vi "niDTS BT INSTR TX UTIL DataType and Rate.vi"(5 "Packet type":T2=enum."DH1", 7 "Data Rate":i32=1) -> (6 "Packet":T1={"PacketType"=enum."DH1", "PacketPayloadDatarate"=1})   [LabVIEW 2015, in "niDTS BT.lvlib" / "niDTS BT INSTR TX.lvclass"]
uses:
  niDTS BT INSTR TX.lvclass
  Includes/niDTS BT INC Packet Type.ctl
  niDTS BT.lvlib
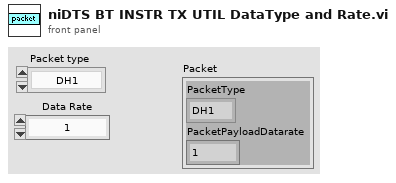
[diagram p1: front panel]
types:
  T1 = cluster{"PacketType":enum16{"DH1", "DH3", "DH5", "LETP"}, "PacketPayloadDatarate":i32}
  T2 = typedef "niDTS BT.lvlib/niDTS BT INC Packet Type.ctl" = enum16{"NULL", "POLL", "FHS", "DM1", "DH1", "HV1", "HV2", "HV3", "EV3", "DV", "AUX1", "DM3", "DH3", "EV4", "EV5", "DM5", "DH5", "LE-TP"}
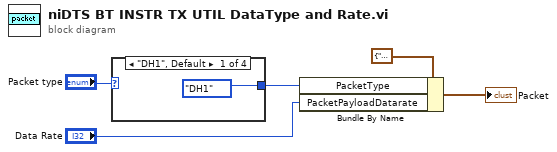
[diagram p0: block diagram]
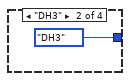
[diagram p2: hidden frame]
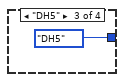
[diagram p3: hidden frame]
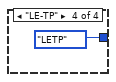
[diagram p4: hidden frame]
diagram:
  n1 = case shown="\"DH1\", Default" "Packet type" {
    tunnel: [enum16{"DH1", "DH3", "DH5", "LETP"}."DH1" ("PacketType") enum16{"DH1", "DH3", "DH5", "LETP"}."DH3" ("PacketType") enum16{"DH1", "DH3", "DH5", "LETP"}."DH5" ("PacketType") enum16{"DH1", "DH3", "DH5", "LETP"}."LETP" ("PacketType")] -> w2
    frame "DH1", Default {
    }
    frame "DH3" {
    }
    frame "DH5" {
    }
    frame "LE-TP" {
    }
  }
  n2 = Bundle By Name(cluster=T1 {"PacketType"=enum."DH1", "PacketPayloadDatarate"=1} ("Packet"), "PacketType"=w2, "PacketPayloadDatarate"="Data Rate") -> (→"Packet":T1)
